vi "Handle Faults.vi"(8 "error in":errorcluster, 9 "Fault":errorcluster, 10 "Device":string, 11 "Fault Monitor in":refnum<class "Fault Monitor.lvclass">) -> (0 "error out":errorcluster, 3 "Fault Monitor out":refnum<class "Fault Monitor.lvclass">)   [LabVIEW 2023, in "Fault Monitor.lvlib" / "Fault Monitor.lvclass"]
uses:
  Library/Fault Monitor.lvclass
  Library/Fault Monitor.lvclass/Fault Monitor.ctl
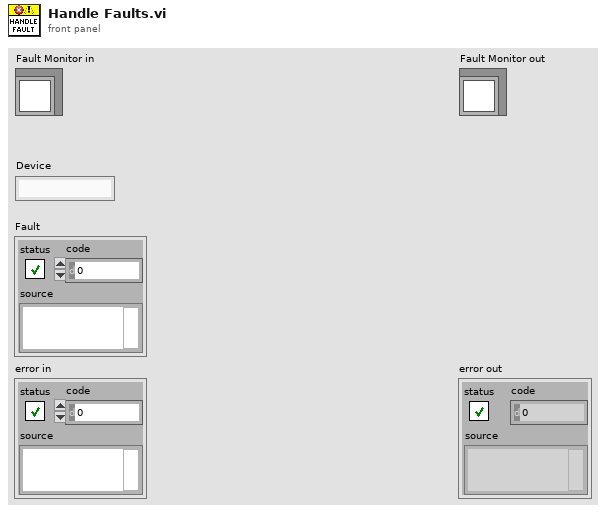
[diagram p1: front panel]
types:
  T1 = typedef "Fault Monitor.lvlib/Fault Monitor.lvclass/Fault Map.ctl" = map{string, errorcluster[]}
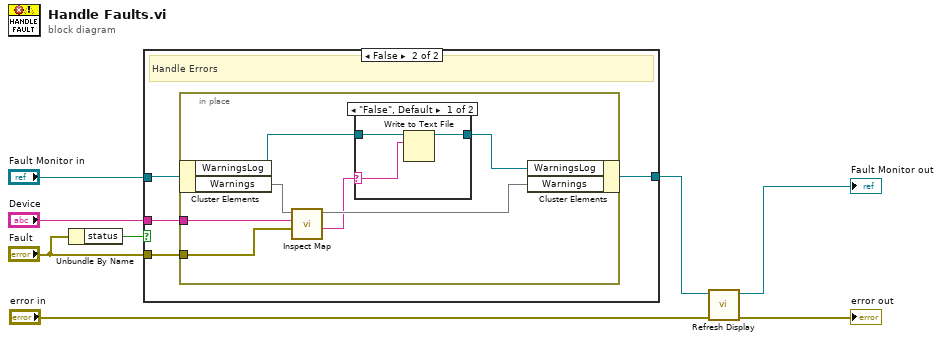
[diagram p0: block diagram]
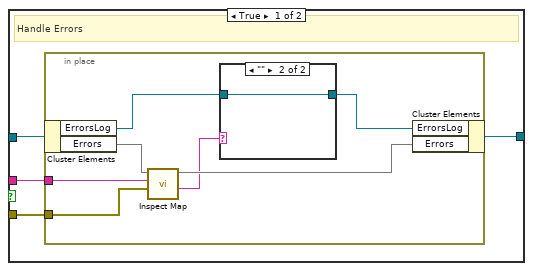
[diagram p2: hidden frame]
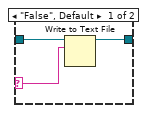
[diagram p3: hidden frame]
diagram:
  n1 = Unbundle By Name("Fault") -> ("status"=w5:bool)
  n2 = case shown="False" w5 {
    tunnel: "Fault Monitor in" -> [w12 w27]
    tunnel: [w11 w26] -> w3
    tunnel: "Device" -> [w10 w25]
    tunnel: "Fault" -> [w9 w24]
    frame True {
      # "Handle Errors"
      n3 = in-place {
        in-place-border: w10 -> [w17]
        in-place-border: w9 -> [w16]
        n4 = in-place-cluster #1(w12) -> ("ErrorsLog"=w14:refnum<file>, "Errors"=w19:map{string, errorcluster[]})
        n5 = call "Inspect Map.vi"("Fault"=w16, "Device"=w17, "Fault map in"=w19) -> ("Log Record"=w15:string, "Fault Map out"=w18:T1)  [unwired: 7 in]
        n6 = case shown="\"\"" w15 {
          selector: w15 -> [w21 _]
          tunnel: w14 -> [w22 w23]
          tunnel: [w20 w23] -> w13
          frame "False", Default {
            n7 = Write to Text File(file (use dialog)=w22, text=w21) -> (refnum out=w20:refnum<file>)  [unwired: 2 in, 2 out]
          }
          frame "" {
          }
        }
        n8 = in-place-cluster #1("ErrorsLog"=w13, "Errors"=w18) -> (w11:refnum<class "Fault Monitor.lvclass">)
      }
    }
    frame False {
      # "Handle Errors"
      n9 = in-place {
        in-place-border: w25 -> [w32]
        in-place-border: w24 -> [w31]
        n10 = in-place-cluster #2(w27) -> ("WarningsLog"=w29:refnum<file>, "Warnings"=w34:map{string, errorcluster[]})
        n11 = call "Inspect Map.vi"("Fault"=w31, "Device"=w32, "Fault map in"=w34) -> ("Log Record"=w30:string, "Fault Map out"=w33:T1)  [unwired: 7 in]
        n12 = case shown="\"False\", Default" w30 {
          selector: w30 -> [w36 _]
          tunnel: w29 -> [w37 w38]
          tunnel: [w35 w38] -> w28
          frame "False", Default {
            n13 = Write to Text File(file (use dialog)=w37, text=w36) -> (refnum out=w35:refnum<file>)  [unwired: 2 in, 2 out]
          }
          frame "" {
          }
        }
        n14 = in-place-cluster #2("WarningsLog"=w28, "Warnings"=w33) -> (w26:refnum<class "Fault Monitor.lvclass">)
      }
    }
  }
  n15 = call "Refresh Display.vi"("error in (no error)"="error in", "Fault Monitor in"=w3) -> ("error out"=→"error out":errorcluster, "Fault Monitor out"=→"Fault Monitor out":refnum<class "Fault Monitor.lvclass">)  [unwired: 8 in]
